vi "Generate Nodes Item.vi"(8 "error in (no error)":errorcluster, 9 "Tree Item In":T1, 10 "Root Tag In":string, 11 "Composite Tree Data in":refnum<class "Composite Tree Data.lvclass">) -> (0 "error out":errorcluster, 1 "Nodes Item Out":T1[](array[typedef]), 3 "Composite Tree Data out":refnum<class "Composite Tree Data.lvclass">)   [LabVIEW 2024, in "Composite Tree Data.lvclass"]
uses:
  Composite Tree Data.lvclass
  Tree/Type Def/Tree Item.ctl
  Composite Tree Data.lvclass/Composite Tree Data.ctl
  Polymorphic VIs/Tree Converter/BFS Index To Tag.vi
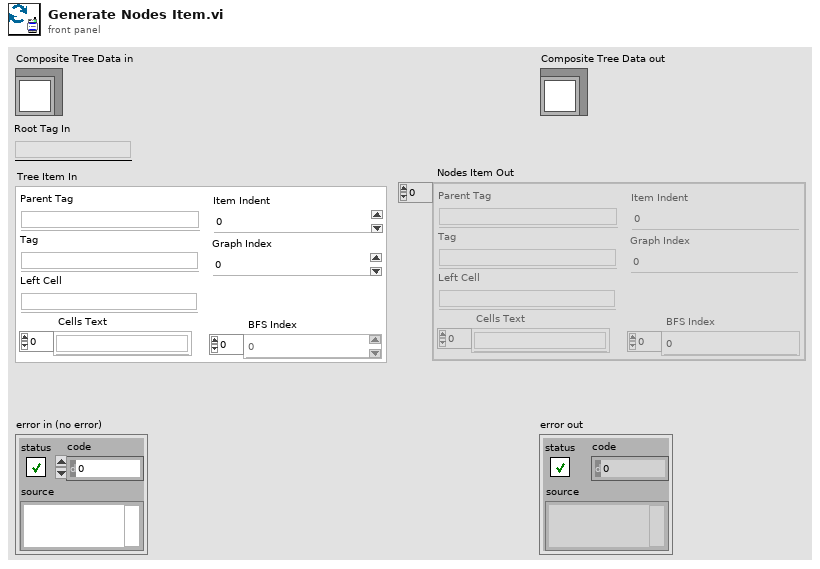
[diagram p1: front panel]
types:
  T1 = typedef "Tree Item.ctl" = cluster{"Parent Tag":string, "Tag":string, "Left Cell":string, "Cells Text":string[], "BFS Index":i32[], "Graph Index":i32, "Item Indent":i32}
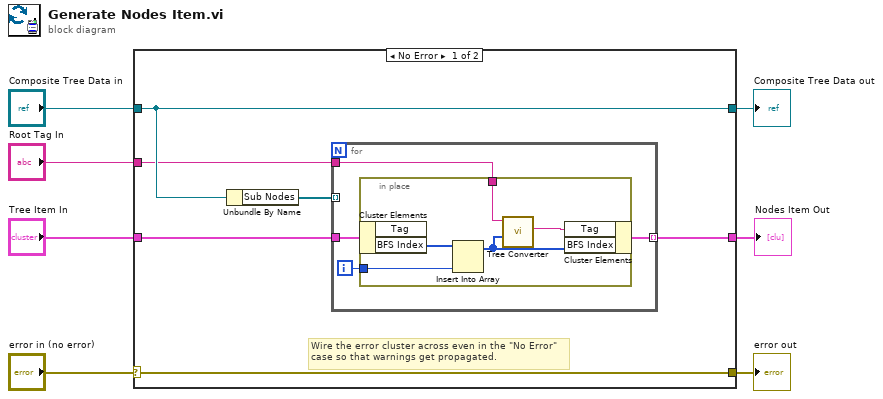
[diagram p0: block diagram]
diagram:
  n1 = case shown="No Error" "error in (no error)" {
    selector: "error in (no error)" -> [w13 w24]
    tunnel: [w13 w24] -> w6
    tunnel: [w9 w23] -> w4
    tunnel: "Composite Tree Data in" -> [w9 w23]
    tunnel: [w11 _] -> w3
    tunnel: "Tree Item In" -> [w10 _]
    tunnel: "Root Tag In" -> [w8 _]
    frame No Error {
      # "Wire the error cluster across even in the \"No Error\"\ncase so that warnings get propagated."
      n2 = Unbundle By Name(w9) -> ("Sub Nodes"=w12:refnum<class "Tree Data.lvclass">[])
      n3 = for {
        tunnel: w12 -> [_] mode=indexing
        tunnel: [w15] -> w11 mode=indexing
        tunnel: w10 -> [w17]
        tunnel: w8 -> [w14]
        i -> [w16]
        n4 = in-place {
          in-place-border: w16 -> [w21]
          in-place-border: w14 -> [w18]
          n5 = in-place-cluster #1(w17) -> ("BFS Index"=w22:i32[])  [unwired: 1 out]
          n6 = Insert Into Array(array=w22, new element=w21) -> (w19:i32[])  [unwired: 1 in]
          n7 = call-poly "Tree Converter.vi"("BFS Index In"=w19, "Root Tag In"=w18) -> ("Tag Out"=w20:string)  [unwired: 9 in]
          n8 = in-place-cluster #1("Tag"=w20, "BFS Index"=w19) -> (w15:T1)
        }
      }
    }
    frame Error {
    }
  }
  "error out" <- w6
  "Composite Tree Data out" <- w4
  "Nodes Item Out" <- w3
